vi "Make Measurement.vi"(6 "Full Waveform":bool, 7 "Record Result (True)":bool, 8 "error in (no error)":errorcluster, 9 "Position":u32, 10 "Channel":string, 11 "Driver Test in":refnum<class "Driver Test.lvclass">) -> (0 "error out":errorcluster, 3 "Value":dbl)   [LabVIEW 2015, in "Driver Test.lvclass"]
uses:
  Driver Test.lvclass
  Measurement Type -- Enum.ctl
  <vilib>/regexp/Match Regular Expression.xnode
  Test Class/Test Class.lvclass
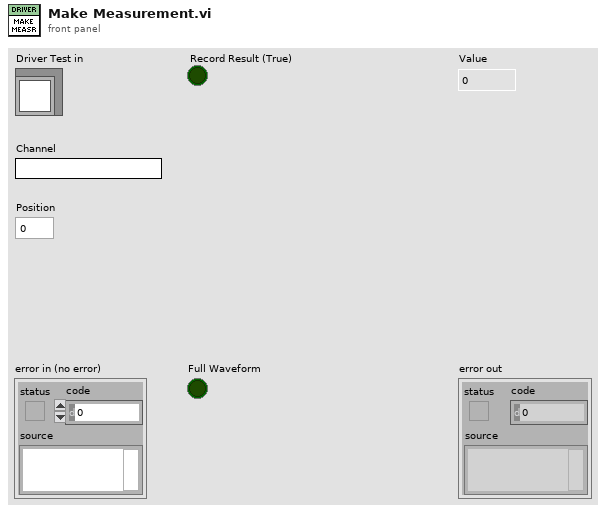
[diagram p1: front panel]
types:
  T1 = typedef "Driver Test.lvclass/Measurement Type -- Enum.ctl" = enum16{"DPM", "DAQmx", "ACPS Voltage", "ACPS Current", "ACPS Power", "DCPS Voltage", "DCPS Current", "DCPS Power"}
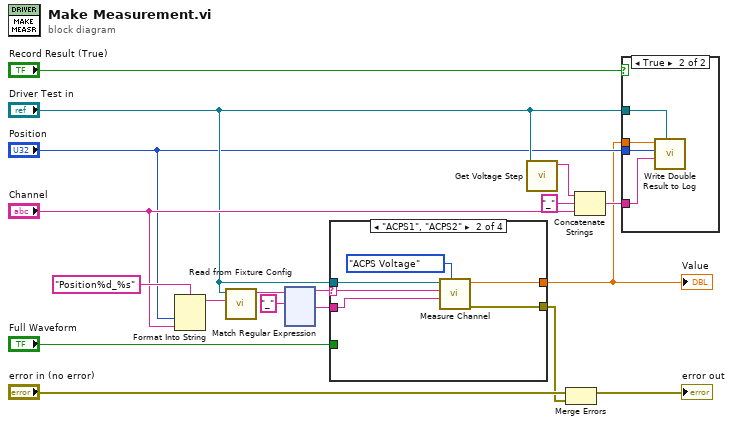
[diagram p0: block diagram]
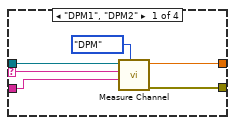
[diagram p3: hidden frame]
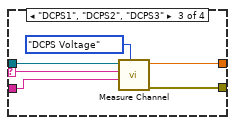
[diagram p4: hidden frame]
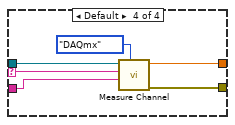
[diagram p5: hidden frame]
diagram:
  n1 = Format Into String(format string="Position%d_%s", "Position", "Channel") -> (resulting string=w15:string)  [unwired: 2 in, 1 out]
  n2 = call-dynamic "Read from Fixture Config.vi"("Key"=w15, "Test Class in"="Driver Test in") -> ("Instrument Info"=w16:string)  [unwired: 8 in, 1 out]
  n3 = xnode "Match Regular Expression"("input string"=w16, "regular expression"="_") -> ("before match"=w14:string, "after match"=w12:string)  [unwired: 4 in, 3 out]
  n4 = case shown="\"ACPS1\", \"ACPS2\"" w14 {
    selector: w14 -> [w23 w29 w35 w41]
    tunnel: w12 -> [w22 w28 w34 w40]
    tunnel: "Driver Test in" -> [w21 w27 w33 w39]
    tunnel: [w20 w26 w32 w38] -> w2
    tunnel: "Full Waveform" -> [_ _ _ _]
    tunnel: [w19 w25 w31 w37] -> w9
    frame "DPM1", "DPM2" {
      n5 = call "Measure Channel.vi"("Measurement Type"=Measurement_Type_--_Enum."DPM", "Channel"=w22, "Instrument"=w23, "Driver Test in"=w21) -> ("error out"=w19:errorcluster, "Measurement"=w20:dbl)  [unwired: 5 in, 1 out]
    }
    frame "ACPS1", "ACPS2" {
      n6 = call "Measure Channel.vi"("Measurement Type"=Measurement_Type_--_Enum."ACPS Voltage", "Channel"=w28, "Instrument"=w29, "Driver Test in"=w27) -> ("error out"=w25:errorcluster, "Measurement"=w26:dbl)  [unwired: 5 in, 1 out]
    }
    frame "DCPS1", "DCPS2", "DCPS3" {
      n7 = call "Measure Channel.vi"("Measurement Type"=Measurement_Type_--_Enum."DCPS Voltage", "Channel"=w34, "Instrument"=w35, "Driver Test in"=w33) -> ("error out"=w31:errorcluster, "Measurement"=w32:dbl)  [unwired: 5 in, 1 out]
    }
    frame Default {
      n8 = call "Measure Channel.vi"("Measurement Type"=Measurement_Type_--_Enum."DAQmx", "Channel"=w40, "Instrument"=w41, "Driver Test in"=w39) -> ("error out"=w37:errorcluster, "Measurement"=w38:dbl)  [unwired: 5 in, 1 out]
    }
  }
  "Value" <- w2
  n9 = call "Get Voltage Step.vi"("Driver Test in"="Driver Test in") -> ("Voltage Step"=w6:string)  [unwired: 9 in, 1 out]
  n10 = Merge Errors("error in (no error)", w9) -> (→"error out":errorcluster)
  n11 = Concatenate Strings(w6, "_" ("string"), "Channel") -> (w5:string)
  n12 = case shown="True" "Record Result (True)" {
    tunnel: w5 -> [_ w46]
    tunnel: "Driver Test in" -> [_ w45]
    tunnel: "Position" -> [_ w44]
    tunnel: w2 -> [_ w43]
    frame False {
    }
    frame True {
      n13 = call "Write Double Result to Log.vi"("Test Class in"=w45, "Label"=w46, "Position"=w44, "Value"=w43) -> ()  [unwired: 7 in, 1 out]
    }
  }
